vi "Read_configuration_2ws.vi"(1 "configuration file path":path) -> (0 "output cluster":T1)   [LabVIEW 2015]
uses:
  <vilib>/LabVIEW Targets/FPGA/cRIO/shared/nicrio_ModuleControls/nicrio_cRIO-9234_DataRatesRing2.ctl
  <vilib>/Utility/config.llb/Read Key (Double).vi
  <vilib>/Utility/config.llb/Read Key (String).vi
  <vilib>/Utility/config.llb/Read Key (U32).vi
  <vilib>/Utility/config.llb/Read Key (Boolean).vi
  <vilib>/Utility/config.llb/NI_LVConfig.lvlib
panel:
  # "ID = 1"
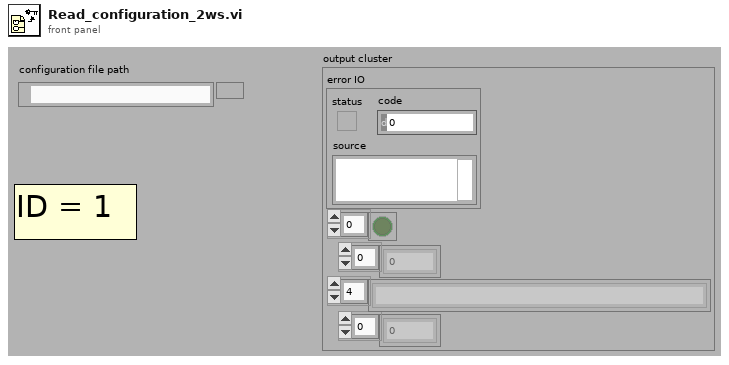
[diagram p1: front panel]
types:
  T1 = cluster{"error IO":errorcluster, bool[], u32[], string[], dbl[]}
  T2 = typedef "nicrio_cRIO-9234_DataRatesRing2.ctl" = u8
  T3 = typedef "NI_LVConfig.lvlib/Config Data RefNum.ctl" = refnum<k1>
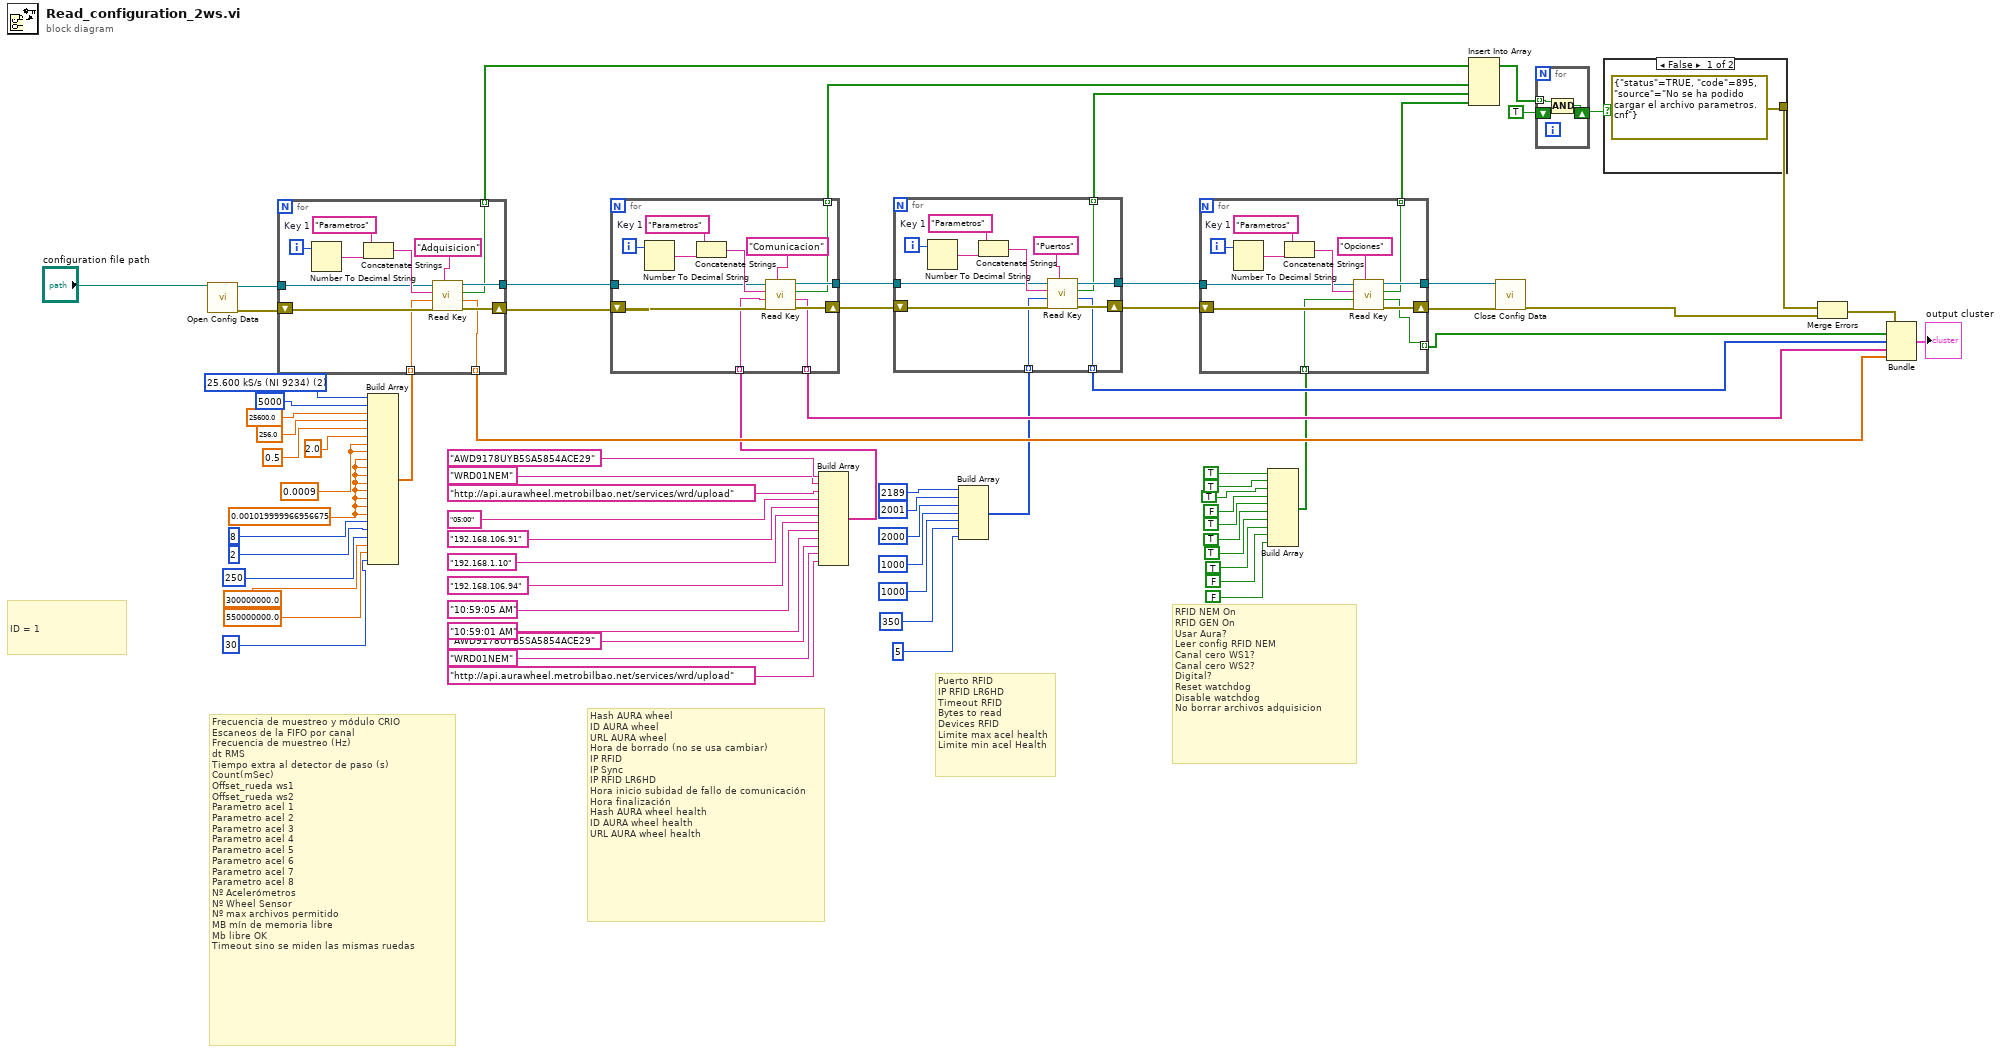
[diagram p0: block diagram]
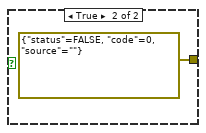
[diagram p2: hidden frame]
diagram:
  w28 = T2 2 items=["51.200 kS/s (NI 9234)"=1, "25.600 kS/s (NI 9234)"=2, "17.067 kS/s (NI 9234)"=3, "12.800 kS/s (NI 9234)"=4, "10.240 kS/s (NI 9234)"=5, "8.533 kS/s (NI 9234)"=6, "7.314 kS/s (NI 9234)"=7, "6.400 kS/s (NI 9234)"=8, "5.689 kS/s (NI 9234)"=9, "5.120 kS/s (NI 9234)"=10, "4.654 kS/s (NI 9234)"=11, "4.267 kS/s (NI 9234)"=12, "3.938 kS/s (NI 9234)"=13, "3.657 kS/s (NI 9234)"=14, "3.413 kS/s (NI 9234)"=15, "3.200 kS/s (NI 9234)"=16, "3.012 kS/s (NI 9234)"=17, "2.845 kS/s (NI 9234)"=18, "2.695 kS/s (NI 9234)"=19, "2.560 kS/s (NI 9234)"=20, "2.438 kS/s (NI 9234)"=21, "2.328 kS/s (NI 9234)"=22, "2.226 kS/s (NI 9234)"=23, "2.133 kS/s (NI 9234)"=24, "2.048 kS/s (NI 9234)"=25, "1.969 kS/s (NI 9234)"=26, "1.896 kS/s (NI 9234)"=27, "1.829 kS/s (NI 9234)"=28, "1.765 kS/s (NI 9234)"=29, "1.707 kS/s (NI 9234)"=30, "1.652 kS/s (NI 9234)"=31] ("Data Rate")
  w9 = 0.0009 ("element")
  w27 = sgl 0.00102
  # "RFID NEM On\nRFID GEN On\nUsar Aura?\nLeer config RFID NEM\nCanal cero WS1?\nCanal cero WS2?\nDigital?\nReset watchdog\nDisable watchdog\nNo borrar archivos adquisicion"
  # "Puerto RFID\nIP RFID LR6HD\nTimeout RFID\nBytes to read\nDevices RFID\nLimite max acel health\nLimite min acel Health"
  # "Hash AURA wheel\nID AURA wheel\nURL AURA wheel\nHora de borrado (no se usa cambiar)\nIP RFID\nIP Sync\nIP RFID LR6HD\nHora inicio subidad de fallo de comunicación\nHora finalización\nHash AURA wheel health\nID AURA wheel health\nURL AURA wheel health"
  # "Frecuencia de muestreo y módulo CRIO\nEscaneos de la FIFO por canal\nFrecuencia de muestreo (Hz)\ndt RMS\nTiempo extra al detector de paso (s)\nCount(mSec)\nOffset_rueda ws1\nOffset_rueda ws2\nParametro acel 1\nParametro acel 2\nParametro acel 3\nParametro acel 4\nParametro acel 5\nParametro acel 6\nParametro acel 7\nParametro acel 8\nNº Acelerómetros\nNº Wheel Sensor\nNº max archivos permitido\nMB mín de memoria libre\nMb libre OK\nTimeout sino se miden las mismas ruedas"
  # "ID = 1"
  n1 = call <vilib>:"Open Config Data.vi"("configuration file path"="configuration file path") -> ("error out"=w45:errorcluster, "refnum"=w46:T3)  [unwired: 2 in, 7 out]
  n2 = Build Array(w28, 5000, 25600.0 ("element"), 256.0 ("element"), 0.5 ("element"), 2.0 ("element"), w9, w9, w27, w27, w27, w27, w27, w27, w27, w27, 8, 2, 250, 300000000.0, 550000000.0, 30) -> (w55:dbl[])
  n3 = for {
    tunnel: w46 -> [w80]
    shift-right: [w78] -> w41
    shift-left: w45 -> [w79]
    tunnel: [w77] -> w42
    tunnel: [w76] -> w73 mode=indexing
    tunnel: [w75] -> w44 mode=indexing
    tunnel: w55 -> [w74] mode=indexing
    i -> [w84]
    w82 = "Parametros"  # Key 1
    n4 = Number To Decimal String(number=w84) -> (decimal integer string=w83:string)  [unwired: 1 in]
    n5 = Concatenate Strings(w82, w83) -> (w81:string)
    n6 = call-poly <vilib>:"Read Key.vi"("section"="Adquisicion", "error in (no error)"=w79, "default value"=w74, "key"=w81, "refnum"=w80) -> ("error out"=w78:errorcluster, "value"=w76:dbl, "found?"=w75:bool, "refnum out"=w77:T3)  [unwired: 3 in]
  }
  n7 = Build Array("AWD9178UYB5SA5854ACE29" ("URL LOGIN"), "WRD01NEM" ("URL ENVÍO PARAM"), "http://api.aurawheel.metrobilbao.net/services/wrd/upload" ("URL LOGOUT"), "05:00", "192.168.106.91" ("element"), "192.168.1.10" ("Time Server\nIP Address"), "192.168.106.94" ("Time Server\nIP Address"), "10:59:05 AM" ("element"), "10:59:01 AM" ("element"), "AWD9178UYB5SA5854ACE29" ("URL LOGIN"), "WRD01NEM" ("URL ENVÍO PARAM"), "http://api.aurawheel.metrobilbao.net/services/wrd/upload" ("URL LOGOUT")) -> (w54:string[])
  n8 = for {
    tunnel: w42 -> [w92]
    shift-right: [w90] -> w64
    shift-left: w41 -> [w91]
    tunnel: [w89] -> w63
    tunnel: [w88] -> w72 mode=indexing
    tunnel: [w87] -> w40 mode=indexing
    tunnel: w54 -> [w86] mode=indexing
    i -> [w96]
    w94 = "Parametros"  # Key 1
    n9 = Number To Decimal String(number=w96) -> (decimal integer string=w95:string)  [unwired: 1 in]
    n10 = Concatenate Strings(w94, w95) -> (w93:string)
    n11 = call-poly <vilib>:"Read Key.vi"("section"="Comunicacion", "error in (no error)"=w91, "default value"=w86, "key"=w93, "refnum"=w92) -> ("error out"=w90:errorcluster, "value"=w88:string, "found?"=w87:bool, "refnum out"=w89:T3)  [unwired: 3 in]
  }
  n12 = Build Array(u16 2189 ("element"), u16 2001 ("element"), u16 2000 ("element"), u16 1000 ("element"), u16 1000 ("element"), u16 350 ("element"), u16 5 ("element")) -> (w53:u16[])
  n13 = for {
    tunnel: w63 -> [w104]
    shift-right: [w102] -> w66
    shift-left: w64 -> [w103]
    tunnel: [w101] -> w65
    tunnel: [w100] -> w71 mode=indexing
    tunnel: [w99] -> w39 mode=indexing
    tunnel: w53 -> [w98] mode=indexing
    i -> [w108]
    w106 = "Parametros"  # Key 1
    n14 = Number To Decimal String(number=w108) -> (decimal integer string=w107:string)  [unwired: 1 in]
    n15 = Concatenate Strings(w106, w107) -> (w105:string)
    n16 = call-poly <vilib>:"Read Key.vi"("section"="Puertos", "error in (no error)"=w103, "default value"=w98, "key"=w105, "refnum"=w104) -> ("error out"=w102:errorcluster, "value"=w100:u32, "found?"=w99:bool, "refnum out"=w101:T3)  [unwired: 3 in]
  }
  n17 = Build Array(TRUE, TRUE, TRUE, FALSE ("element"), TRUE ("element"), TRUE ("element"), TRUE ("element"), TRUE ("element"), FALSE ("element"), FALSE ("element")) -> (w50:bool[])
  n18 = for {
    tunnel: w65 -> [w116]
    shift-right: [w114] -> w67
    shift-left: w66 -> [w115]
    tunnel: [w113] -> w68
    tunnel: [w112] -> w70 mode=indexing
    tunnel: [w111] -> w38 mode=indexing
    tunnel: w50 -> [w110] mode=indexing
    i -> [w120]
    w118 = "Parametros"  # Key 1
    n19 = Number To Decimal String(number=w120) -> (decimal integer string=w119:string)  [unwired: 1 in]
    n20 = Concatenate Strings(w118, w119) -> (w117:string)
    n21 = call-poly <vilib>:"Read Key.vi"("section"="Opciones", "error in (no error)"=w115, "default value"=w110, "key"=w117, "refnum"=w116) -> ("error out"=w114:errorcluster, "value"=w112:bool, "found?"=w111:bool, "refnum out"=w113:T3)  [unwired: 3 in]
  }
  n22 = Insert Into Array(array=w44, new element #1=w40, new element #2=w39, new element #3=w38) -> (w47:bool[])  [unwired: 1 in]
  n23 = call <vilib>:"Close Config Data.vi"("error in (no error)"=w67, "refnum"=w68) -> ("error out"=w61:errorcluster)  [unwired: 8 in, 1 out]
  n24 = for {
    shift-right: [w123] -> w48
    shift-left: TRUE -> [w124]
    tunnel: w47 -> [w122] mode=indexing
    n25 = Compound Arithmetic op=AND(w122, w124) -> (w123:bool)
  }
  n26 = case shown="False" w48 {
    tunnel: [errorcluster {"status"=TRUE, "code"=895, "source"="No se ha podido cargar el archivo parametros.cnf"} ("error out") errorcluster {"status"=FALSE, "code"=0, "source"=""} ("error out")] -> w62
    frame False {
    }
    frame True {
    }
  }
  n27 = Merge Errors(w62, w61) -> (w60:errorcluster)
  n28 = Bundle("error IO"=w60, w70, w71, w72, w73) -> (→"output cluster":T1)  [unwired: 1 in]
